vi "arm_update.vi"(0 "j2":dbl, 1 "j1":dbl, 5 "j3":dbl, 7 "j4":dbl, 9 "j5":dbl, 11 "j6":dbl, 12 "element":dbl, 13 "kinematic parameters":T1[](array[typedef])) -> (4 "SceneObject out":refnum<vi>, 6 "end effector transform":T3)   [LabVIEW 2019]
uses:
  <vilib>/Analysis/Matrix/Datatypes/RealMatrix.ctl
  <vilib>/robotics/Kinematics/DH Kinematic Parameters.ctl
  <vilib>/robotics/Kinematics/Link/Joint Type.ctl
  <vilib>/robotics/Kinematics/Analytical/Initialize Generic Serial Arm.vi
  <vilib>/robotics/Kinematics/Robot/Forward Kinematics (Point).vi
  <vilib>/robotics/Kinematics/Analytical/NI_Robotics_AnalyticKinematics.lvlib
  <vilib>/robotics/Kinematics/Robot/NI_Robotics_Serial Robot Arm.lvclass
  <vilib>/robotics/Kinematics/Plotting/NI_Robotics_3DKinematics.lvlib
  <vilib>/robotics/Kinematics/NI_Kinematics.lvlib
  <vilib>/Analysis/Matrix/NI_Matrix.lvlib
  <vilib>/robotics/Kinematics/Link/NI_Robotics_Link.lvclass
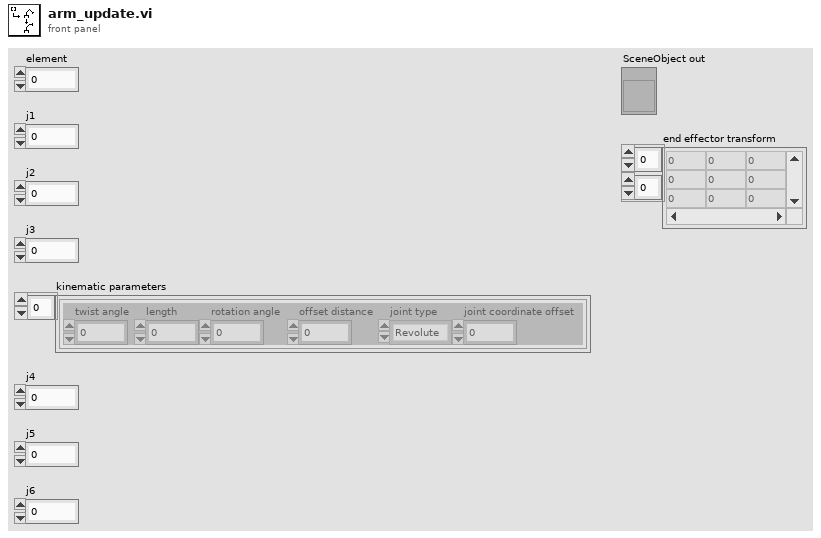
[diagram p1: front panel]
types:
  T1 = typedef "DH Kinematic Parameters.ctl" = cluster{"twist angle":dbl, "length":dbl, "rotation angle":dbl, "offset distance":dbl, "joint type":T2, "joint coordinate offset":dbl}
  T2 = typedef "NI_Robotics_Link.lvclass/Joint Type.ctl" = enum16{"Revolute", "Prismatic"}
  T3 = typedef "NI_Matrix.lvlib/RealMatrix.ctl" = dbl[][]
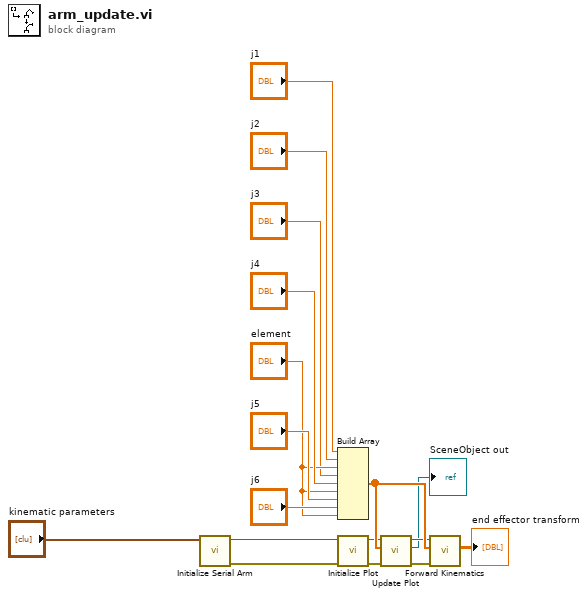
[diagram p0: block diagram]
diagram:
  n1 = call-poly <vilib>:"Initialize Serial Arm.vi"("kinematic parameters"="kinematic parameters") -> ("error out"=w2:errorcluster, "serial arm out"=w3:refnum<class "NI_Robotics_Serial Robot Arm.lvclass">)  [unwired: 9 in]
  n2 = Build Array("j1", "j2", "element", "j3", "j4", "element", "j5", "j6", "element") -> (w13:dbl[])
  n3 = call <vilib>:"Initialize Plot.vi"("error in (no error)"=w2, "serial arm in"=w3) -> ("error out"=w8:errorcluster, "serial arm out"=w7:refnum<class "NI_Robotics_Serial Robot Arm.lvclass">)  [unwired: 8 in]
  n4 = call <vilib>:"Update Plot.vi"("error in (no error)"=w8, "joint positions"=w13, "serial arm in"=w7) -> ("error out"=w12:errorcluster, "serial arm scene"=→"SceneObject out":refnum<vi>, "serial arm out"=w11:refnum<class "NI_Robotics_Serial Robot Arm.lvclass">)  [unwired: 6 in]
  n5 = call-poly <vilib>:"Forward Kinematics.vi"("error in (no error)"=w12, "joint positions"=w13, "serial arm in"=w11) -> ("end effector transform"=→"end effector transform":T3)  [unwired: 6 in, 2 out]
